vi "close all relay channel.vi"(8 "error in (no error)":errorcluster, 11 "Relay Indetifier":i32=349111800) -> (0 "error out":errorcluster, 3 "Relay Indetifier Out":i32)   [LabVIEW 2022 SP3, in "usb_relay_device.lvlib"]
doc: "int EXPORT_API usb_relay_device_close_all_relay_channel(int hHandle);"
uses:
  usb_relay_device.lvlib
  AppBuilderFiles/RunTimeExe/data/usb_relay_device.dll
panel:
  out "function return":i32
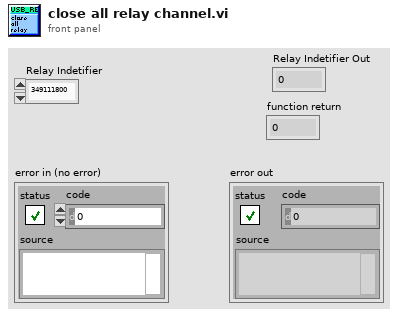
[diagram p1: front panel]
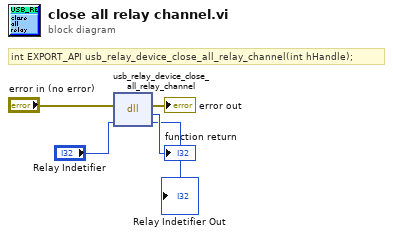
[diagram p0: block diagram]
diagram:
  # "int EXPORT_API usb_relay_device_close_all_relay_channel(int hHandle);"
  n1 = dll-call lib="D:/LabVIEWSuite_64_OS/AppBuilderFiles/RunTimeExe/data/usb_relay_device.*" fn="usb_relay_device_close_all_relay_channel"(error in="error in (no error)", "hHandle"="Relay Indetifier") -> (error out=→"error out":errorcluster, →"function return":i32, "hHandle"=→"Relay Indetifier Out":i32)  [unwired: 2 in, 1 out]
